vi "save parameters.vi"() -> ()   [LabVIEW 2014]
uses:
  <vilib>/Utility/config.llb/NI_LVConfig.lvlib
  TIRF Lock/autofocus-globals.vi
panel:
  out "Boolean":bool
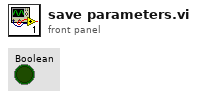
[diagram p1: front panel]
types:
  T1 = enum32{"Invalid", "Standard", "Closed", "Hidden", "Minimized", "Maximized"}
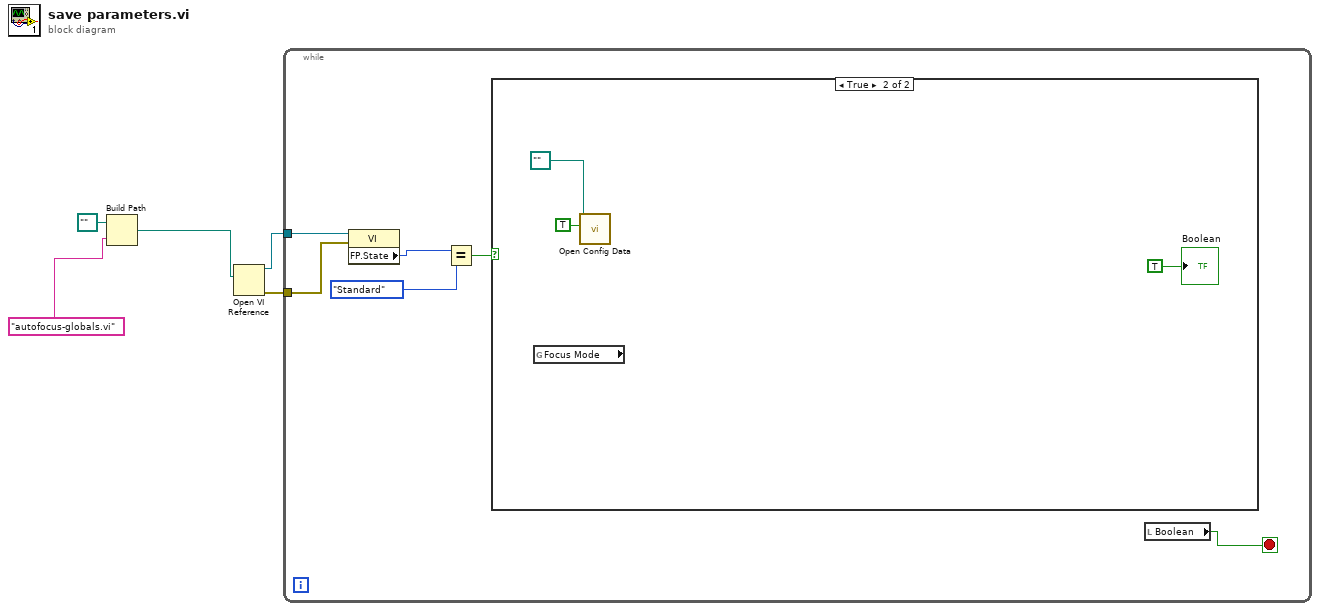
[diagram p0: block diagram]
diagram:
  n1 = Build Path(base path=path "", name or relative path="autofocus-globals.vi") -> (appended path=w4:path)
  n2 = Open VI Reference(vi path=w4) -> (vi reference=w3:refnum<vi>, error out=w2:errorcluster)  [unwired: 1 in, 4 out]
  n3 = while {
    tunnel: w3 -> [w8]
    tunnel: w2 -> [w7]
    stop <- w11 stop-if-true
    n4 = property class="VI"(reference=w8, error in=w7) -> ("FP.State"=w9:T1)  [unwired: 2 out]
    n5 = Equal?(x=w9, y=T1."Standard") -> (x = y?=w6:bool)
    n6 = case shown="True" w6 {
      frame False {
      }
      frame True {
        n7 = global read "autofocus-globals.vi" "Focus Mode"() -> ()  [unwired: 1 out]
        n8 = call <vilib>:"Open Config Data.vi"("create file if necessary (T)"=TRUE, "configuration file path"=path "") -> ()  [unwired: 1 in, 9 out]
        "Boolean" <- TRUE
      }
    }
    n9 = local read "Boolean"() -> (w11:bool)
  }
